vi "Execution_Message_BuildLogMessage.vi"(8 "error in (no error)":errorcluster, 11 "ProcessStartedMessage in":refnum<class "ProcessStartedMessage.lvclass">) -> (0 "error out":errorcluster, 3 "ProcessStartedMessage out":refnum<class "ProcessStartedMessage.lvclass">)   [LabVIEW 2013, in "ProcessStartedMessage.lvclass"]
uses:
  ProcessStartedMessage.lvclass
  Messages.lvclass
  ProcessStartedMessage.lvclass/ProcessStartedMessage.ctl
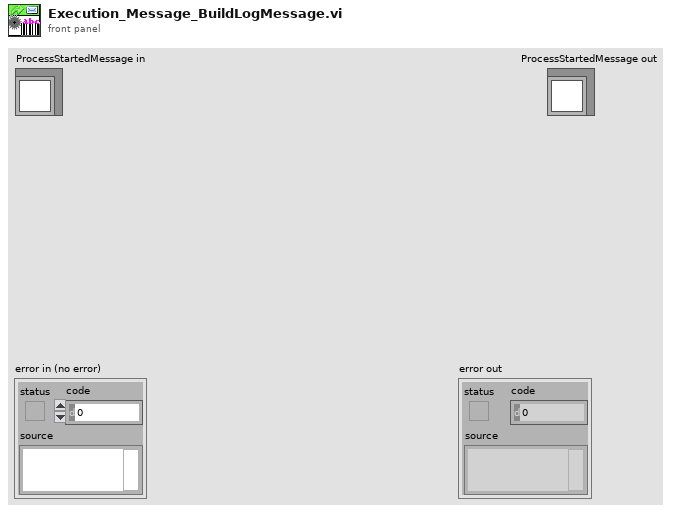
[diagram p1: front panel]
types:
  T1 = typedef "ProcessStartedMessage.lvclass/ProcessStartState.ctl" = enum16{"Started", "Started with error"}
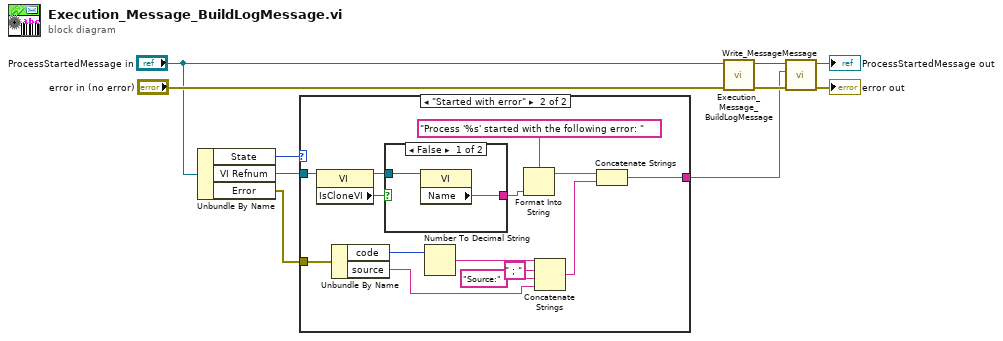
[diagram p0: block diagram]
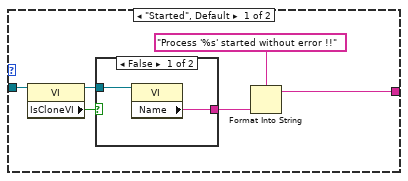
[diagram p2: hidden frame]
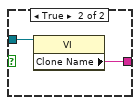
[diagram p3: hidden frame]
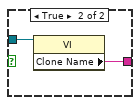
[diagram p4: hidden frame]
diagram:
  n1 = Unbundle By Name("ProcessStartedMessage in") -> ("State"=w4:T1, "VI Refnum"=w3:refnum<vi>, "Error"=w2:errorcluster)
  n2 = case shown="\"Started with error\"" w4 {
    tunnel: w3 -> [w15 w31]
    tunnel: w2 -> [_ w22]
    tunnel: [w11 w28] -> w1
    frame "Started", Default {
      n3 = property class="VI"(reference=w15) -> (reference out=w13:refnum<vi>, "IsCloneVI"=w14:bool)  [unwired: 1 in, 1 out]
      n4 = case shown="False" w14 {
        tunnel: w13 -> [w18 w20]
        tunnel: [w17 w19] -> w12
        frame False {
          n5 = property class="VI"(reference=w18) -> ("Name"=w17:string)  [unwired: 1 in, 2 out]
        }
        frame True {
          n6 = property class="VI"(reference=w20) -> ("Clone Name"=w19:string)  [unwired: 1 in, 2 out]
        }
      }
      n7 = Format Into String(format string="Process '%s' started without error !!", w12) -> (resulting string=w11:string)  [unwired: 2 in, 1 out]
    }
    frame "Started with error" {
      n8 = property class="VI"(reference=w31) -> (reference out=w33:refnum<vi>, "IsCloneVI"=w34:bool)  [unwired: 1 in, 1 out]
      n9 = Unbundle By Name(w22) -> ("code"=w23:i32, "source"=w27:string)
      n10 = case shown="False" w34 {
        tunnel: w33 -> [w36 w38]
        tunnel: [w35 w37] -> w32
        frame False {
          n11 = property class="VI"(reference=w36) -> ("Name"=w35:string)  [unwired: 1 in, 2 out]
        }
        frame True {
          n12 = property class="VI"(reference=w38) -> ("Clone Name"=w37:string)  [unwired: 1 in, 2 out]
        }
      }
      n13 = Number To Decimal String(number=w23) -> (decimal integer string=w24:string)  [unwired: 1 in]
      n14 = Format Into String(format string="Process '%s' started with the following error: ", w32) -> (resulting string=w29:string)  [unwired: 2 in, 1 out]
      n15 = Concatenate Strings(w24, " ; " ("string"), "Source:" ("string"), w27) -> (w21:string)
      n16 = Concatenate Strings(w29, w21) -> (w28:string)
    }
  }
  n17 = call-parent "Execution_Message_BuildLogMessage.vi"("error in (no error)"="error in (no error)", "Messages in"="ProcessStartedMessage in") -> ("error out"=w7:errorcluster, "Messages out"=w9:refnum<class "ProcessStartedMessage.lvclass">)  [unwired: 8 in]
  n18 = call-dynamic "Write_MessageMessage.vi"("error in (no error)"=w7, "Message"=w1, "Messages in"=w9) -> ("error out"=→"error out":errorcluster, "Messages out"=→"ProcessStartedMessage out":refnum<class "ProcessStartedMessage.lvclass">)  [unwired: 7 in]
